vi "Close MeasurementLink Session.vi"(8 "error in":errorcluster, 9 "initialize and close session behavior":T1, 10 "session in":variant, 11 "session factory in":refnum<class "NI-DMM.lvclass">) -> (0 "error out":errorcluster)   [LabVIEW 2020, in "NI-DMM.lvclass"]
doc: "Closes the local session. If the session represents a remote session, <b>initialize and close session behavior</b> determines whether closing the local session closes the server session or detaches from the server session."
uses:
  NI-DMM.lvclass
  <vilib>/MeasurementLink/MeasurementLink Instrument/ISession Factory/Initialize and Close Session Behavior.ctl
  NI-DMM.lvclass/NI-DMM.ctl
  <vilib>/MeasurementLink/MeasurementLink Instrument/ISession Factory/ISession Factory.lvclass
  <instrlib>/niDMM/nidmm.llb/niDMM Close.vi
  <instrlib>/niDMM/nidmm.llb/niDMM Detach gRPC Session.vi
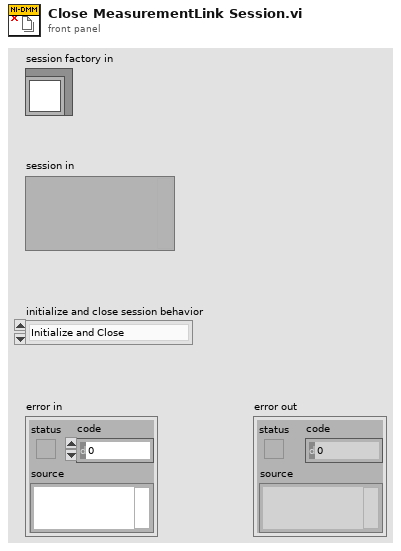
[diagram p1: front panel]
types:
  T1 = typedef "MeasurementLink Instrument.lvlib/ISession Factory.lvclass/Initialize and Close Session Behavior.ctl" = enum16{"Initialize and Close", "Attach and Detach", "Initialize and Detach", "Attach and Close"}
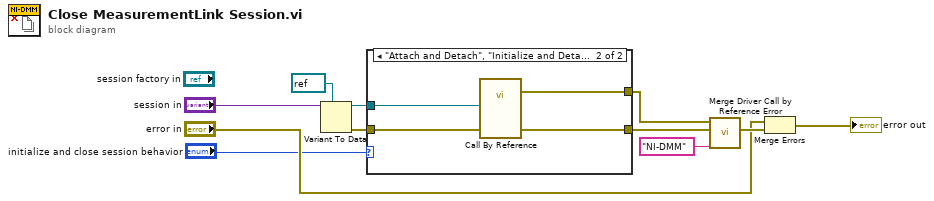
[diagram p0: block diagram]
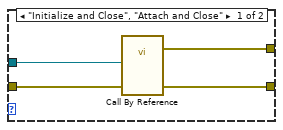
[diagram p2: hidden frame]
diagram:
  n1 = Variant To Data(type=refnum<k15> refnum ("instrument handle"), Variant="session in") -> (data=w10:refnum<k15>, error out=w11:errorcluster)  [unwired: 1 in]
  n2 = case shown="\"Attach and Detach\", \"Initialize and Detach\"" "initialize and close session behavior" {
    tunnel: w11 -> [w15 w19]
    tunnel: w10 -> [w14 w17]
    tunnel: [w13 w18] -> w7
    tunnel: [w12 w16] -> w6
    frame "Initialize and Close", "Attach and Close" {
      n3 = call-by-ref "?"("error in (no error)"=w15, "instrument handle"=w14) -> (error out=w12:errorcluster, 0:"error out"=w13:errorcluster)  [unwired: 11 in, 1 out]
    }
    frame "Attach and Detach", "Initialize and Detach" {
      n4 = call-by-ref "?"("error in (no error)"=w19, "instrument handle"=w17) -> (error out=w16:errorcluster, 0:"error out"=w18:errorcluster)  [unwired: 11 in, 1 out]
    }
  }
  n5 = call <vilib>:"Merge Driver Call by Reference Error.vi"("driver name"="NI-DMM", "called vi error"=w7, "call by ref error"=w6) -> ("error out"=w5:errorcluster)  [unwired: 8 in]
  n6 = Merge Errors("error in", w5) -> (→"error out":errorcluster)
